vi "VoltageInputStart.vi"(0 "Device Info":T1={"Serial Number"=-1, "Channel"=0, "Port"=0}, 1 "Data Interval":i32=-1, 2 "Change Trigger":dbl, 3 "Power Supply":i32(ring)=2 items=["POWER_SUPPLY_OFF"=1, "POWER_SUPPLY_12V"=2, "POWER_SUPPLY_24V"=3], 5 "IsHubPort":bool, 7 "Range":u32(ring)=11 caption="Voltage Range" items=["VOLTAGE_RANGE_10mV"=1, "VOLTAGE_RANGE_40mV"=2, "VOLTAGE_RANGE_200mV"=3, "VOLTAGE_RANGE_312_5mV"=4, "VOLTAGE_RANGE_400mV"=5, "VOLTAGE_RANGE_1000mV"=6, "VOLTAGE_RANGE_2V"=7, "VOLTAGE_RANGE_5V"=8, "VOLTAGE_RANGE_15V"=9, "VOLTAGE_RANGE_40V"=10, "VOLTAGE_RANGE_AUTO"=11], 9 "Sensor Type":u32(ring) items=["SENSOR_TYPE_VOLTAGE"=0, "SENSOR_TYPE_1114"=11140, "SENSOR_TYPE_1117"=11170, "SENSOR_TYPE_1123"=11230, "SENSOR_TYPE_1127"=11270, "SENSOR_TYPE_1130_PH"=11301, "SENSOR_TYPE_1130_ORP"=11302, "SENSOR_TYPE_1132"=11320, "SENSOR_TYPE_1133"=11330, "SENSOR_TYPE_1135"=11350, "SENSOR_TYPE_1142"=11420, "SENSOR_TYPE_1143"=11430, "SENSOR_TYPE_3500"=35000, "SENSOR_TYPE_3501"=35010, "SENSOR_TYPE_3502"=35020, "SENSOR_TYPE_3503"=35030, "SENSOR_TYPE_3507"=35070, "SENSOR_TYPE_3508"=35080, "SENSOR_TYPE_3509"=35090, "SENSOR_TYPE_3510"=35100, "SENSOR_TYPE_3511"=35110, "SENSOR_TYPE_3512"=35120, "SENSOR_TYPE_3513"=35130, "SENSOR_TYPE_3514"=35140, "SENSOR_TYPE_3515"=35150, "SENSOR_TYPE_3516"=35160, "SENSOR_TYPE_3517"=35170, "SENSOR_TYPE_3518"=35180, "SENSOR_TYPE_3519"=35190, "SENSOR_TYPE_3584"=35840, "SENSOR_TYPE_3585"=35850, "SENSOR_TYPE_3586"=35860, "SENSOR_TYPE_3587"=35870, "SENSOR_TYPE_3588"=35880, "SENSOR_TYPE_3589"=35890, "SENSOR_TYPE_ADP1000_PH"=110000, "SENSOR_TYPE_ADP1000_ORP"=110001], 11 "error in (no error)":errorcluster, 12 "Connection":u16(ring) items=["No Preference", "Remote", "Local"], 13 "Timeout (mSec)":i32=5000) -> (4 "Phidget ID":u64, 6 "Serial Number Return":i32, 10 "Attached?":bool, 15 "error out":errorcluster)   [LabVIEW 2012, in "Phidget Voltage Input.lvlib"]
doc: "${VoltageInput:StartHeader}"
uses:
  <instrlib>/Phidgets/Phidget Voltage Input/Phidget Voltage Input.lvlib
  <instrlib>/Phidgets/Phidget Common/Phidget Common.lvlib
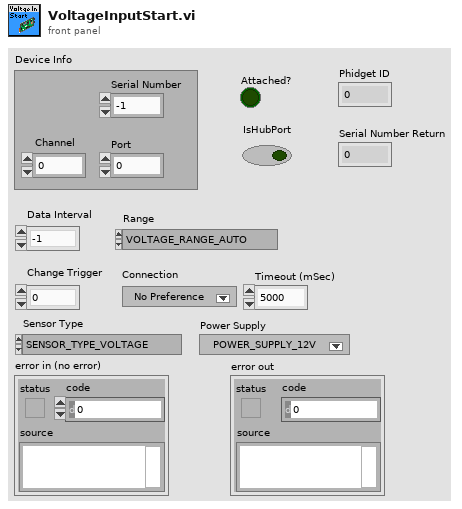
[diagram p1: front panel]
types:
  T1 = cluster{"Serial Number":i32, "Channel":i32, "Port":i32}
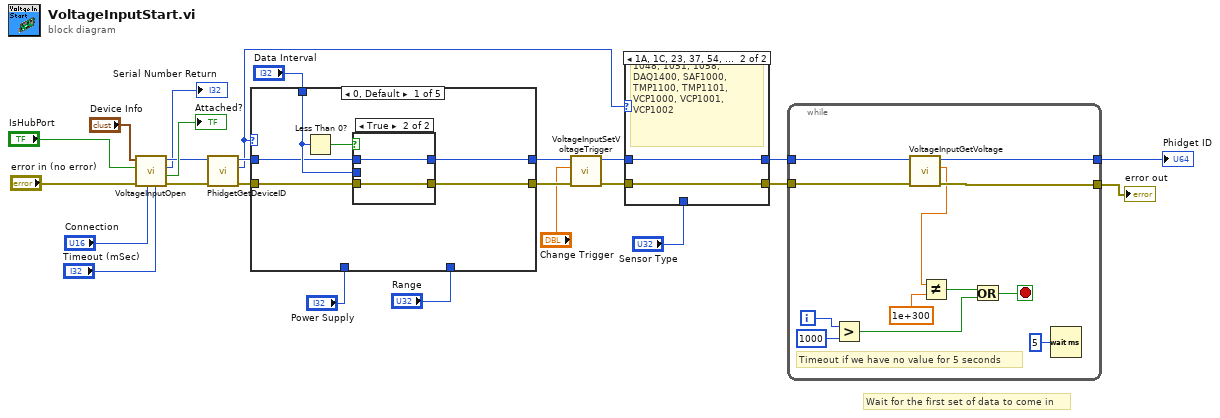
[diagram p0: block diagram]
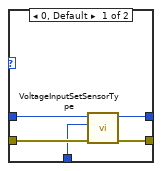
[diagram p2: hidden frame]
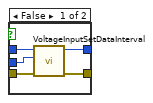
[diagram p3: hidden frame]
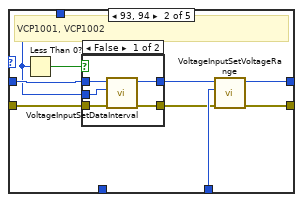
[diagram p4: hidden frame]
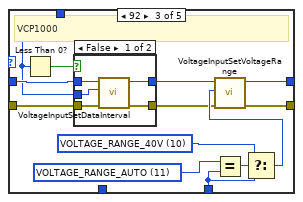
[diagram p6: hidden frame]
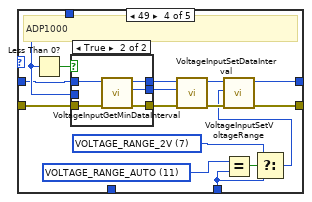
[diagram p8: hidden frame]
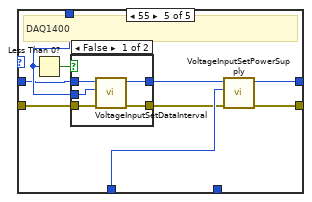
[diagram p10: hidden frame]
diagram:
  # "Wait for the first set of data to come in"
  n1 = call <instrlib>:"VoltageInputOpen.vi"("Timeout (mSec)"="Timeout (mSec)", "Connection"="Connection", "error in"="error in (no error)", "IsHubPort"="IsHubPort", "Device Info"="Device Info") -> ("error out"=w22:errorcluster, "Attached?"=→"Attached?":bool, "Serial Number Return"=→"Serial Number Return":i32, "Phidget ID"=w21:u64)  [unwired: 3 in]
  n2 = call <instrlib>:"PhidgetGetDeviceID.vi"("error in (no error)"=w22, "Device In"=w21) -> ("error out"=w19:errorcluster, "Devie IDs"=w3:u32, "Device Out"=w20:u64)  [unwired: 6 in]
  n3 = case shown="0, Default" w3 {
    tunnel: w19 -> [w31 w44 w60 w85 w105]
    tunnel: [w27 w46 w67 w82 w104] -> w15
    tunnel: w20 -> [w29 w43 w59 w80 w102]
    tunnel: [w28 w45 w66 w81 w103] -> w16
    tunnel: "Data Interval" -> [w30 w42 w57 w86 w106]
    tunnel: "Range" -> [_ w47 w62 w76 _]
    tunnel: "Power Supply" -> [_ _ _ _ w101]
    frame 0, Default {
      n4 = Less Than 0?(x=w30) -> (x < 0?=w26:bool)
      n5 = case shown="True" w26 {
        tunnel: w29 -> [w36 w38]
        tunnel: w31 -> [w34 w37]
        tunnel: [w33 w38] -> w28
        tunnel: [w32 w37] -> w27
        tunnel: w30 -> [w35 _]
        frame False {
          n6 = call <instrlib>:"VoltageInputSetDataInterval.vi"("error in (no error)"=w34, "Interval"=w35, "Device In"=w36) -> ("error out"=w32:errorcluster, "Device Out"=w33:u64)  [unwired: 6 in]
        }
        frame True {
        }
      }
    }
    frame 93, 94 {
      # "VCP1001, VCP1002"
      n7 = Less Than 0?(x=w42) -> (x < 0?=w39:bool)
      n8 = case shown="False" w39 {
        tunnel: w43 -> [w52 w54]
        tunnel: w44 -> [w50 w53]
        tunnel: [w49 w54] -> w41
        tunnel: [w48 w53] -> w40
        tunnel: w42 -> [w51 _]
        frame False {
          n9 = call <instrlib>:"VoltageInputSetDataInterval.vi"("error in (no error)"=w50, "Interval"=w51, "Device In"=w52) -> ("error out"=w48:errorcluster, "Device Out"=w49:u64)  [unwired: 6 in]
        }
        frame True {
        }
      }
      n10 = call <instrlib>:"VoltageInputSetVoltageRange.vi"("error in (no error)"=w40, "Voltage Range"=w47, "Device In"=w41) -> ("error out"=w46:errorcluster, "Device Out"=w45:u64)  [unwired: 6 in]
    }
    frame 92 {
      w63 = u32 10 items=["VOLTAGE_RANGE_10mV"=1, "VOLTAGE_RANGE_40mV"=2, "VOLTAGE_RANGE_200mV"=3, "VOLTAGE_RANGE_312_5mV"=4, "VOLTAGE_RANGE_400mV"=5, "VOLTAGE_RANGE_1000mV"=6, "VOLTAGE_RANGE_2V"=7, "VOLTAGE_RANGE_5V"=8, "VOLTAGE_RANGE_15V"=9, "VOLTAGE_RANGE_40V"=10, "VOLTAGE_RANGE_AUTO"=11] ("Range")
      w65 = u32 11 items=["VOLTAGE_RANGE_10mV"=1, "VOLTAGE_RANGE_40mV"=2, "VOLTAGE_RANGE_200mV"=3, "VOLTAGE_RANGE_312_5mV"=4, "VOLTAGE_RANGE_400mV"=5, "VOLTAGE_RANGE_1000mV"=6, "VOLTAGE_RANGE_2V"=7, "VOLTAGE_RANGE_5V"=8, "VOLTAGE_RANGE_15V"=9, "VOLTAGE_RANGE_40V"=10, "VOLTAGE_RANGE_AUTO"=11] ("Range")
      # "VCP1000"
      n11 = Less Than 0?(x=w57) -> (x < 0?=w58:bool)
      n12 = case shown="False" w58 {
        tunnel: w59 -> [w72 w74]
        tunnel: w60 -> [w70 w73]
        tunnel: [w69 w74] -> w56
        tunnel: [w68 w73] -> w55
        tunnel: w57 -> [w71 _]
        frame False {
          n13 = call <instrlib>:"VoltageInputSetDataInterval.vi"("error in (no error)"=w70, "Interval"=w71, "Device In"=w72) -> ("error out"=w68:errorcluster, "Device Out"=w69:u64)  [unwired: 6 in]
        }
        frame True {
        }
      }
      n14 = Equal?(x=w65, y=w62) -> (x = y?=w64:bool)
      n15 = Select(t=w63, s=w64, f=w62) -> (s? t:f=w61:u32)
      n16 = call <instrlib>:"VoltageInputSetVoltageRange.vi"("error in (no error)"=w55, "Voltage Range"=w61, "Device In"=w56) -> ("error out"=w67:errorcluster, "Device Out"=w66:u64)  [unwired: 6 in]
    }
    frame 49 {
      w77 = u32 7 items=["VOLTAGE_RANGE_10mV"=1, "VOLTAGE_RANGE_40mV"=2, "VOLTAGE_RANGE_200mV"=3, "VOLTAGE_RANGE_312_5mV"=4, "VOLTAGE_RANGE_400mV"=5, "VOLTAGE_RANGE_1000mV"=6, "VOLTAGE_RANGE_2V"=7, "VOLTAGE_RANGE_5V"=8, "VOLTAGE_RANGE_15V"=9, "VOLTAGE_RANGE_40V"=10, "VOLTAGE_RANGE_AUTO"=11] ("Range")
      w79 = u32 11 items=["VOLTAGE_RANGE_10mV"=1, "VOLTAGE_RANGE_40mV"=2, "VOLTAGE_RANGE_200mV"=3, "VOLTAGE_RANGE_312_5mV"=4, "VOLTAGE_RANGE_400mV"=5, "VOLTAGE_RANGE_1000mV"=6, "VOLTAGE_RANGE_2V"=7, "VOLTAGE_RANGE_5V"=8, "VOLTAGE_RANGE_15V"=9, "VOLTAGE_RANGE_40V"=10, "VOLTAGE_RANGE_AUTO"=11] ("Range")
      # "ADP1000"
      n17 = Less Than 0?(x=w86) -> (x < 0?=w87:bool)
      n18 = case shown="True" w87 {
        tunnel: w80 -> [w92 w98]
        tunnel: w85 -> [w91 w97]
        tunnel: [w92 w96] -> w89
        tunnel: [w91 w95] -> w88
        tunnel: [w93 w94] -> w90
        tunnel: w86 -> [w93 _]
        frame False {
        }
        frame True {
          n19 = call <instrlib>:"VoltageInputGetMinDataInterval.vi"("error in (no error)"=w97, "Device In"=w98) -> ("error out"=w95:errorcluster, "Min Data Interval"=w94:i32, "Device Out"=w96:u64)  [unwired: 6 in]
        }
      }
      n20 = call <instrlib>:"VoltageInputSetDataInterval.vi"("error in (no error)"=w88, "Interval"=w90, "Device In"=w89) -> ("error out"=w84:errorcluster, "Device Out"=w83:u64)  [unwired: 6 in]
      n21 = Equal?(x=w79, y=w76) -> (x = y?=w78:bool)
      n22 = Select(t=w77, s=w78, f=w76) -> (s? t:f=w75:u32)
      n23 = call <instrlib>:"VoltageInputSetVoltageRange.vi"("error in (no error)"=w84, "Voltage Range"=w75, "Device In"=w83) -> ("error out"=w82:errorcluster, "Device Out"=w81:u64)  [unwired: 6 in]
    }
    frame 55 {
      # "DAQ1400"
      n24 = Less Than 0?(x=w106) -> (x < 0?=w107:bool)
      n25 = case shown="False" w107 {
        tunnel: w102 -> [w112 w114]
        tunnel: w105 -> [w110 w113]
        tunnel: [w109 w114] -> w100
        tunnel: [w108 w113] -> w99
        tunnel: w106 -> [w111 _]
        frame False {
          n26 = call <instrlib>:"VoltageInputSetDataInterval.vi"("error in (no error)"=w110, "Interval"=w111, "Device In"=w112) -> ("error out"=w108:errorcluster, "Device Out"=w109:u64)  [unwired: 6 in]
        }
        frame True {
        }
      }
      n27 = call <instrlib>:"VoltageInputSetPowerSupply.vi"("error in (no error)"=w99, "Power Supply"=w101, "Device In"=w100) -> ("error out"=w104:errorcluster, "Device Out"=w103:u64)  [unwired: 6 in]
    }
  }
  n28 = call <instrlib>:"VoltageInputSetVoltageTrigger.vi"("error in (no error)"=w15, "Trigger"="Change Trigger", "Device In"=w16) -> ("error out"=w7:errorcluster, "Device Out"=w6:u64)  [unwired: 6 in]
  n29 = case shown="1A, 1C, 23, 37, 54, 58, 59, 5C..5E" w3 {
    tunnel: w7 -> [w119 w120]
    tunnel: w6 -> [w118 w121]
    tunnel: [w117 w121] -> w5
    tunnel: [w116 w120] -> w4
    tunnel: "Sensor Type" -> [w115 _]
    frame 0, Default {
      n30 = call <instrlib>:"VoltageInputSetSensorType.vi"("error in (no error)"=w119, "Sensor Type"=w115, "Device In"=w118) -> ("error out"=w116:errorcluster, "Device Out"=w117:u64)  [unwired: 6 in]
    }
    frame 26, 28, 35, 55, 84, 88, 89, 92..94 {
      # "1048, 1051, 1058, DAQ1400, SAF1000, TMP1100, TMP1101, VCP1000, VCP1001, VCP1002"
    }
  }
  n31 = while {
    tunnel: w5 -> [w131]
    tunnel: w4 -> [w130]
    tunnel: [w128] -> w18
    tunnel: [w129] -> w24
    i -> [w126]
    stop <- w123 stop-if-true
    # "Timeout if we have no value for 5 seconds"
    n32 = Greater?(x=w126, y=1000) -> (0:w124:bool)
    n33 = call <instrlib>:"VoltageInputGetVoltage.vi"("error in (no error)"=w130, "Device In"=w131) -> ("error out"=w129:errorcluster, "Votlage"=w122:dbl, "Device Out"=w128:u64)  [unwired: 6 in]
    n34 = Not Equal?(x=w122, y=1e+300) -> (x != y?=w125:bool)
    n35 = Or(x=w125, y=w124) -> (x .or. y?=w123:bool)
    n36 = Wait (ms)(milliseconds to wait=u32 5) -> ()  [unwired: 1 out]
  }
  "error out" <- w24
  "Phidget ID" <- w18
